vi "AutoGoHome.vi"(8 "error in (no error)":errorcluster) -> (0 "error out":errorcluster, 2 "Desired Extend":dbl, 3 "Desired Lift":dbl)   [LabVIEW 2020]
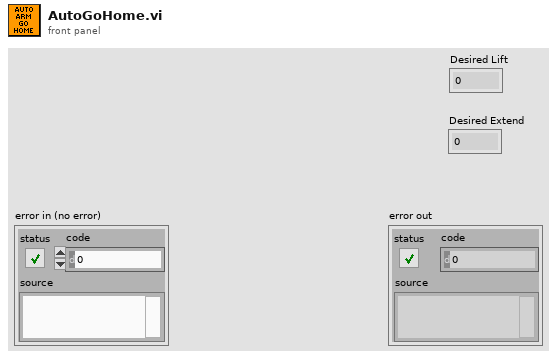
[diagram p1: front panel]
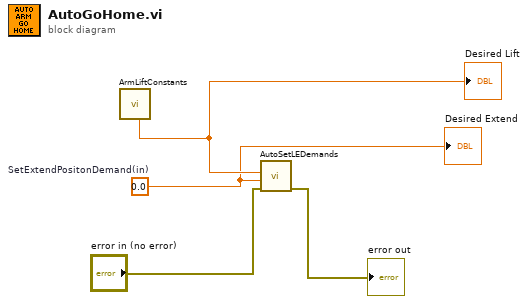
[diagram p0: block diagram]
diagram:
  w1 = 0.0  # SetExtendPositonDemand(in)
  n1 = call "ArmLiftConstants.vi"() -> ("Default Angle"=w2:dbl)  [unwired: 8 in, 3 out]
  "Desired Lift" <- w2
  n2 = call "AutoSetLEDemands.vi"("error in (no error)"="error in (no error)", "SetExtendPositonDemand(in)"=w1, "SetLIftPostionDemand(d)"=w2) -> ("error out"=→"error out":errorcluster)  [unwired: 8 in]
  "Desired Extend" <- w1
